vi "GetSiblings__slk_tc.vi"(0 "tree control in":refnum<class "TreeControl.lvclass">, 5 "input tag (current tag)":string, 11 "error in (no error)":errorcluster) -> (4 "tree control out":refnum<class "TreeControl.lvclass">, 6 "sibling tags":string[](array[string]), 10 "input tag index":i32, 15 "error out":errorcluster)   [LabVIEW 2020, in "TreeControl.lvclass"]
doc: "Retrieves a 1-D array of tags of all items in the tree that have the same parent and deletes the requested tag giving all siblings of an item. Uses the currently selected item if the tag input is unwired."
uses:
  Library/TreeControl.lvclass
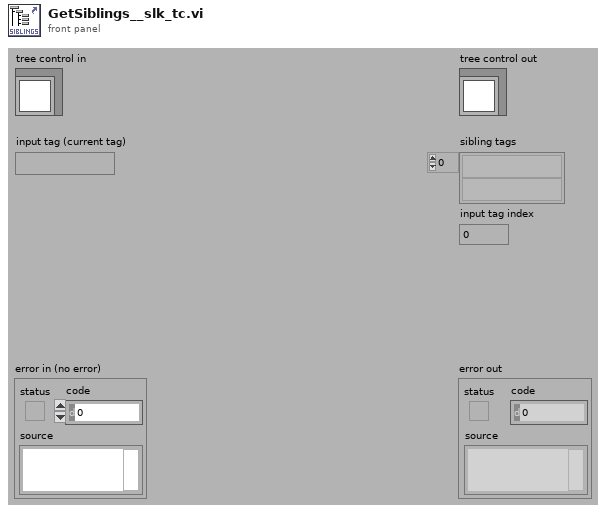
[diagram p1: front panel]
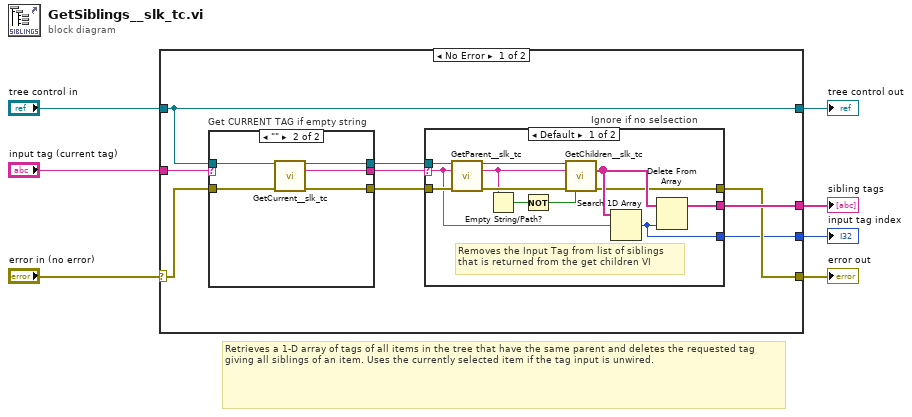
[diagram p0: block diagram]
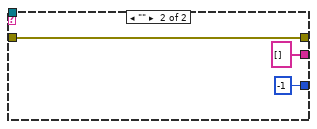
[diagram p2: hidden frame]
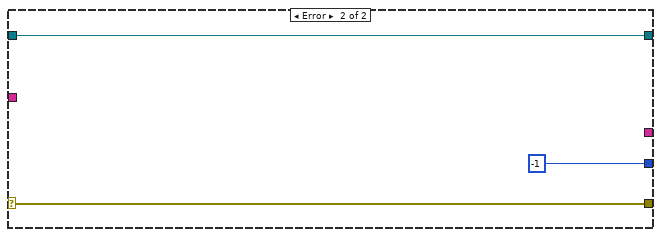
[diagram p4: hidden frame]
diagram:
  # "Retrieves a 1-D array of tags of all items in the tree that have the same parent and deletes the requested tag giving all siblings of an item. Uses the currently selected item if the tag input is unwired."
  n1 = case shown="No Error" "error in (no error)" {
    selector: "error in (no error)" -> [w10 w42]
    tunnel: [w9 w42] -> w6
    tunnel: [w16 w41] -> w4
    tunnel: "tree control in" -> [w16 w41]
    tunnel: "input tag (current tag)" -> [w15 _]
    tunnel: [w11 _] -> w2
    tunnel: [w8 -1 ("index of element")] -> w1
    frame No Error {
      n2 = case "Get CURRENT TAG if empty string" shown="\"\"" w15 {
        selector: w15 -> [w34 _]
        tunnel: [w34 w39] -> w14
        tunnel: w16 -> [w32 w38]
        tunnel: w10 -> [w33 w37]
        tunnel: [w33 w36] -> w13
        tunnel: [w32 w35] -> w12
        frame Default {
        }
        frame "" {
          n3 = call "GetCurrent__slk_tc.vi"("tree control in"=w38, "error in (no error)"=w37) -> ("tree control out"=w35:refnum<class "TreeControl.lvclass">, "current tag"=w39:string, "error out"=w36:errorcluster)  [unwired: 1 in, 10 out]
        }
      }
      n4 = case "Ignore if no selsection" shown="Default" w14 {
        selector: w14 -> [w24 _]
        tunnel: w13 -> [w27 w30]
        tunnel: w12 -> [w28 _]
        tunnel: [w22 string[] [] ("Children Tags")] -> w11
        tunnel: [w21 w30] -> w9
        tunnel: [w20 -1 ("index of element")] -> w8
        frame Default {
          # "Removes the Input Tag from list of siblings\nthat is returned from the get children VI"
          n5 = call "GetParent__slk_tc.vi"("tree control in"=w28, "child tag (\"\")"=w24, "error in (no error)"=w27) -> ("tree control out"=w26:refnum<class "TreeControl.lvclass">, "parent tag"=w19:string, "error out"=w25:errorcluster)  [unwired: 10 out]
          n6 = Empty String/Path?(string/path=w19) -> (empty?=w18:bool)
          n7 = Not(x=w18) -> (.not. x?=w17:bool)
          n8 = call "GetChildren__slk_tc.vi"("tree control in"=w26, "parent tag (\"\")"=w19, "error in (no error)"=w25, "use current (T)"=w17) -> ("children tags"=w23:string[], "error out"=w21:errorcluster)  [unwired: 10 out]
          n9 = Search 1D Array(1D array=w23, element=w24) -> (index of element=w20:i32)  [unwired: 1 out]
          n10 = Delete From Array(array=w23, index=w20) -> (array with subset deleted=w22:string[])  [unwired: 1 in, 1 out]
        }
        frame "" {
        }
      }
    }
    frame Error {
    }
  }
  "error out" <- w6
  "tree control out" <- w4
  "sibling tags" <- w2
  "input tag index" <- w1
